vi "Thermometer.vi"(1 "Units (0: Celsius)":u16(ring) items=["Celsius", "Fahrenheit"]) -> (0 "Temperature":dbl(slide) scale=0.0..100.0)   [LabVIEW 2018]
doc: "This VI measures temperature using the temperature sensor on the DAQ BNC-2120 terminal block."
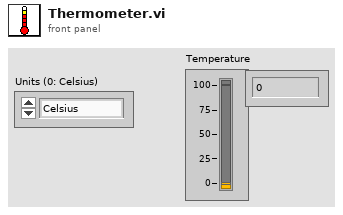
[diagram p1: front panel]
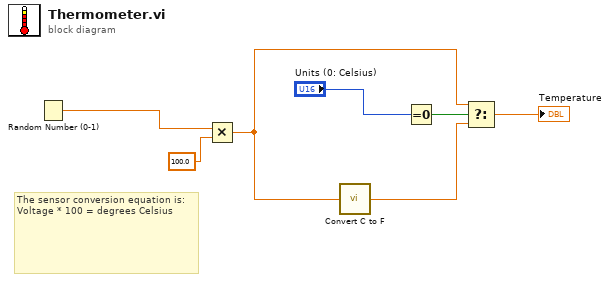
[diagram p0: block diagram]
diagram:
  # "The sensor conversion equation is: \nVoltage * 100 = degrees Celsius"
  n1 = Random Number (0-1)() -> (number: 0 to 1=w1:dbl)
  n2 = Multiply(x=w1, y=100.0) -> (x*y=w6:dbl)
  n3 = call "Convert C to F.vi"("Degrees Celsius"=w6) -> ("Degrees Fahrenheit"=w7:dbl)
  n4 = Equal To 0?(x="Units (0: Celsius)") -> (x = 0?=w2:bool)
  n5 = Select(t=w6, s=w2, f=w7) -> (s? t:f=→"Temperature":dbl)
